vi "Launch Test Station_3(Event Callback).vi"(4 "user event":refnum<user-event>, 5 "Event Data":cluster{"sender":refnum<k24>, "e":refnum<k24>}, 6 "Control Ref":refnum<k24>, 7 "Event Common Data":T1) -> ()   [LabVIEW 2019]
uses:
  System.Windows.Forms
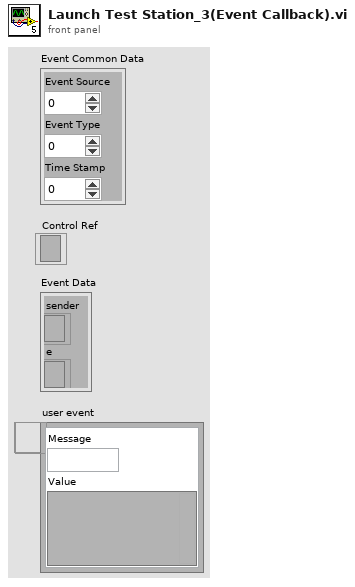
[diagram p1: front panel]
types:
  T1 = cluster{"Event Source":i32, "Event Type":u32, "Time Stamp":u32}
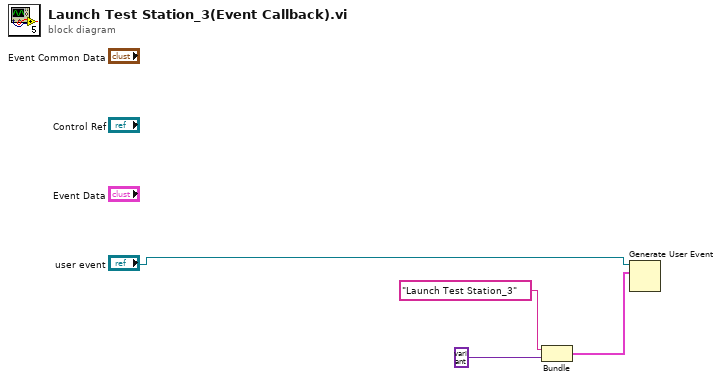
[diagram p0: block diagram]
diagram:
  n1 = Bundle("event data"="Launch Test Station_3", variant) -> (w1:cluster{"event data":string, variant})  [unwired: 1 in]
  n2 = Generate User Event(user event="user event", event data cluster=w1) -> ()  [unwired: 2 in, 2 out]
